vi "FlatToRichgoogle_protobuf_Field.vi"(5 "OutputClusterType":T1, 11 "InputCluster":T6) -> (3 "OutputCluster":T1)   [LabVIEW 2020, in "MeasurementLink Measurement Server Internal.lvlib"]
uses:
  MeasurementLink Measurement Server Internal.lvlib
  google_protobuf_Field_Flat.ctl
  google_protobuf_Field_Kind.ctl
  google_protobuf_Field_Cardinality.ctl
  google_protobuf_Option_Flat.ctl
  google_protobuf_Any_Flat.ctl
  google_protobuf_Field.ctl
  google_protobuf_Option.ctl
  google_protobuf_Any.ctl
  FlatToRichgoogle_protobuf_Any.vi
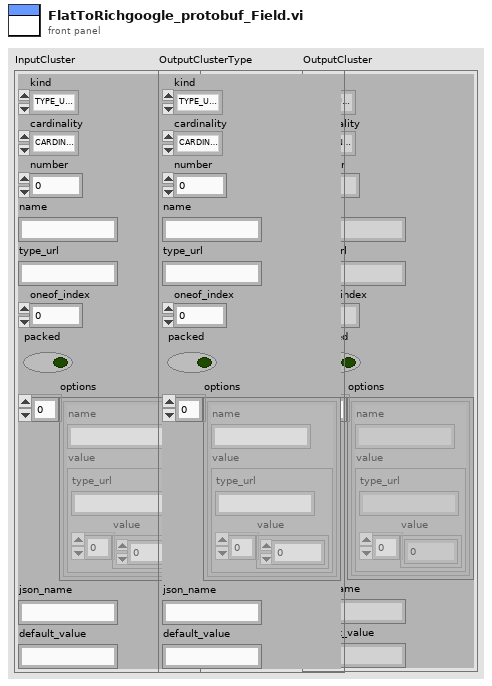
[diagram p1: front panel]
types:
  T1 = typedef "MeasurementLink Measurement Server Internal.lvlib/google_protobuf_Field.ctl" = cluster{"kind":T2, "cardinality":T3, "number":i32, "name":string, "type_url":string, "oneof_index":i32, "packed":bool, "options":T4[], "json_name":string, "default_value":string}
  T2 = typedef "MeasurementLink Measurement Server Internal.lvlib/google_protobuf_Field_Kind.ctl" = enum32{"TYPE_UNKNOWN", "TYPE_DOUBLE", "TYPE_FLOAT", "TYPE_INT64", "TYPE_UINT64", "TYPE_INT32", "TYPE_FIXED64", "TYPE_FIXED32", "TYPE_BOOL", "TYPE_STRING", "TYPE_GROUP", "TYPE_MESSAGE", "TYPE_BYTES", "TYPE_UINT32", "TYPE_ENUM", "TYPE_SFIXED32", "TYPE_SFIXED64", "TYPE_SINT32", "TYPE_SINT64"}
  T3 = typedef "MeasurementLink Measurement Server Internal.lvlib/google_protobuf_Field_Cardinality.ctl" = enum32{"CARDINALITY_UNKNOWN", "CARDINALITY_OPTIONAL", "CARDINALITY_REQUIRED", "CARDINALITY_REPEATED"}
  T4 = typedef "MeasurementLink Measurement Server Internal.lvlib/google_protobuf_Option.ctl" = cluster{"name":string, "value":T5}
  T5 = typedef "MeasurementLink Measurement Server Internal.lvlib/google_protobuf_Any.ctl" = cluster{"type_url":string, "value":u8[]}
  T6 = typedef "MeasurementLink Measurement Server Internal.lvlib/google_protobuf_Field_Flat.ctl" = cluster{"kind":T2, "cardinality":T3, "number":i32, "name":string, "type_url":string, "oneof_index":i32, "packed":bool, "options":T7[], "json_name":string, "default_value":string}
  T7 = typedef "MeasurementLink Measurement Server Internal.lvlib/google_protobuf_Option_Flat.ctl" = cluster{"name":string, "value":T8}
  T8 = typedef "MeasurementLink Measurement Server Internal.lvlib/google_protobuf_Any_Flat.ctl" = cluster{"type_url":string, "value":u8[]}
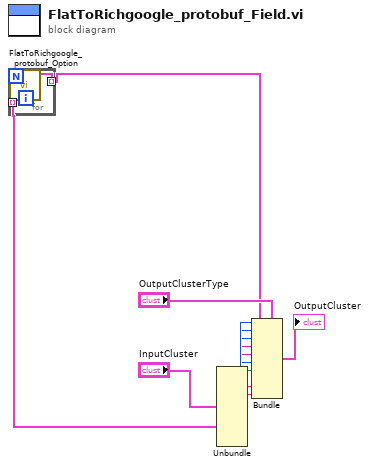
[diagram p0: block diagram]
diagram:
  n1 = Unbundle "Unbundle"("InputCluster") -> ("kind"=w11:T2, "cardinality"=w10:T3, "number"=w9:i32, "name"=w8:string, "type_url"=w7:string, "oneof_index"=w6:i32, "packed"=w5:bool, "options"=w4:T7[], "json_name"=w2:string, "default_value"=w1:string)
  n2 = for {
    tunnel: w4 -> [w16] mode=indexing
    tunnel: [w15] -> w3 mode=indexing
    n3 = call "FlatToRichgoogle_protobuf_Option.vi"("InputCluster"=w16) -> ("OutputCluster"=w15:T4)  [unwired: 10 in]
  }
  n4 = Bundle "Bundle"(cluster="OutputClusterType", "kind"=w11, "cardinality"=w10, "number"=w9, "name"=w8, "type_url"=w7, "oneof_index"=w6, "packed"=w5, "options"=w3, "json_name"=w2, "default_value"=w1) -> (→"OutputCluster":T1)
